vi "new_graph.vi"(4 "CurvesId":i32, 5 "D&T":string, 7 "connection ref":T1) -> (0 "error out":errorcluster, 1 "Waveform Graph":cluster{sgl, sgl, sgl[]}, 2 "reason":string)   [LabVIEW 2010]
uses:
  <vilib>/addons/database/Connection.llb/Conn ObjectReference.ctl
  <vilib>/addons/database/NI_Database_API.lvlib
panel:
  out "resulting string":string
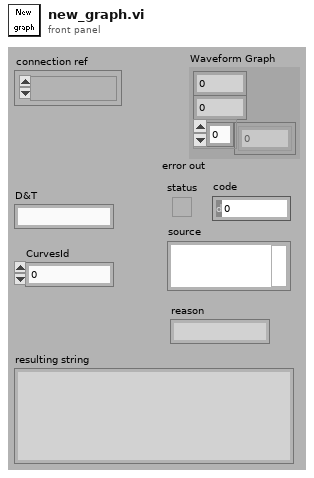
[diagram p1: front panel]
types:
  T1 = typedef "NI_Database_API.lvlib/Conn ObjectReference.ctl" = refnum<k1>
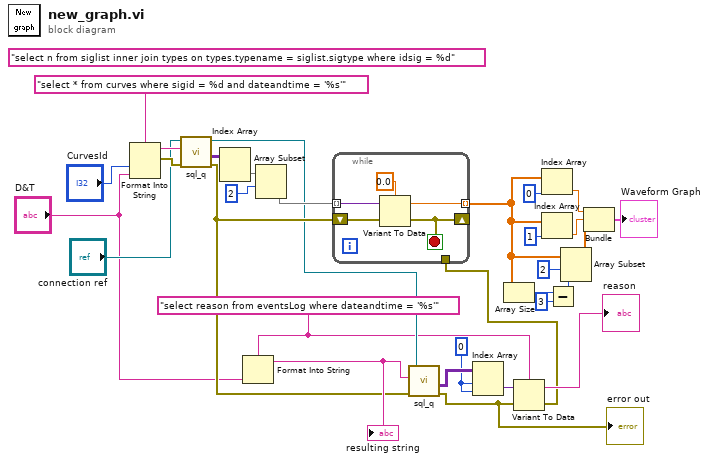
[diagram p0: block diagram]
diagram:
  w5 = 0 ("index (row)")
  w4 = "select reason from eventsLog where dateandtime = '%s'"
  (unwired) "select n from siglist inner join types on types.typename = siglist.sigtype where idsig = %d" ("regular expression (\"\")")
  n1 = Format Into String(format string="select * from curves where sigid = %d and dateandtime = '%s'" ("optional clause"), "CurvesId", "D&T") -> (resulting string=w23:string, error out=w18:errorcluster)  [unwired: 2 in]
  n2 = call "sql_q.vi"("error in"=w18, "SQL query"=w23, "connect ref"="connection ref") -> ("error out"=w10:errorcluster, "recordset data"=w25:variant[][], "conn ref out"=w9:T1)  [unwired: 1 in, 1 out]
  n3 = Index Array(array=w25) -> (element=w26:variant[])  [unwired: 2 in]
  n4 = Format Into String(format string=w4, "D&T") -> (resulting string=w11:string)  [unwired: 2 in, 1 out]
  "resulting string" <- w11
  n5 = Array Subset(array=w26, index=2) -> (w24:variant[])  [unwired: 1 in]
  n6 = call "sql_q.vi"("error in"=w10, "SQL query"=w11, "connect ref"=w9) -> ("error out"=w2:errorcluster, "recordset data"=w7:variant[][])  [unwired: 1 in, 2 out]
  "error out" <- w2
  n7 = Index Array(array=w7, index (row)=w5, index (col)=w5) -> (element=w6:variant)
  n8 = Variant To Data(error in=w2, Variant=w6, type=w4) -> (error out=w1:errorcluster, data=→"reason":string)
  n9 = while {
    tunnel: [w36] -> w14 mode=indexing
    tunnel: w24 -> [w35] mode=indexing
    shift-right: [w33] -> _
    shift-left: w10 -> [w32]
    tunnel: w1 -> [_]
    stop <- w33 stop-if-true
    n10 = Variant To Data(error in=w32, Variant=w35, type=0.0) -> (error out=w33:errorcluster, data=w36:dbl)
  }
  n11 = Array Size(array=w14) -> (size(s)=w15:i32)
  n12 = Index Array(array=w14, index=0 ("disabled index (col)")) -> (element=w21:dbl)
  n13 = Index Array(array=w14, index=1 ("disabled index (col)")) -> (element=w22:dbl)
  n14 = Subtract(x=w15, y=3) -> (x-y=w13:i32)
  n15 = Array Subset(array=w14, index=2, length=w13) -> (w30:dbl[])
  n16 = Bundle(w21, w22, w30) -> (→"Waveform Graph":cluster{dbl, dbl, dbl[]})  [unwired: 1 in]
